vi "Handle Error.vi"(8 "error in (no error)":errorcluster, 11 "CIFPlugin in":refnum<class "Template_Plugin.lvclass">) -> (0 "error out":errorcluster, 3 "CIFPlugin out":refnum<class "Template_Plugin.lvclass">)   [LabVIEW 2021, in "Template_Plugin.lvclass"]
uses:
  Template_Plugin.lvclass
  Template_Plugin.lvclass/Template_Plugin.ctl
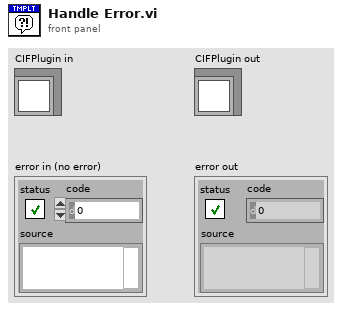
[diagram p1: front panel]
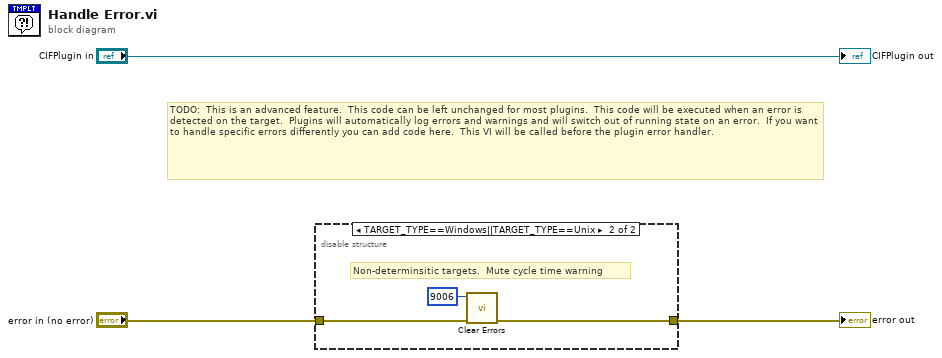
[diagram p0: block diagram]
diagram:
  # "TODO:  This is an advanced feature.  This code can be left unchanged for most plugins.  This code will be executed when an error is detected on the target.  Plugins will automatically log errors and warnings and will switch out of running state on an error.  If you want to handle specific errors differently you can add code here.  This VI will be called before the plugin error handler."
  n1 = disable-structure shown="TARGET_TYPE==Windows||TARGET_TYPE==Unix" {
    disable-tunnel: "error in (no error)" -> [w4 w7]
    disable-tunnel: [w4 w6] -> w1
    frame condition #0 {
    }
    frame condition #1 (active) {
      # "Non-determinsitic targets.  Mute cycle time warning"
      n2 = call <vilib>:"Clear Errors.vi"("error in (no error)"=w7, "specific error code to clear (0: all)"=9006) -> ("error out"=w6:errorcluster)  [unwired: 4 in, 1 out]
    }
  }
  "error out" <- w1
  "CIFPlugin out" <- "CIFPlugin in"
